vi "Get Value.vi"(8 "error in (no error)":errorcluster, 11 "Acquired Result in":refnum<class "Acquired Result.lvclass">) -> (0 "error out":errorcluster, 2 "Value":dynamicdata(graph) caption="Filtered Signal", 3 "Acquired Result out":refnum<class "Acquired Result.lvclass">)   [LabVIEW 2021, in "Acquired Result.lvclass"]
uses:
  Acquired Result.lvclass
  Acquired Result.lvclass/Acquired Result.ctl
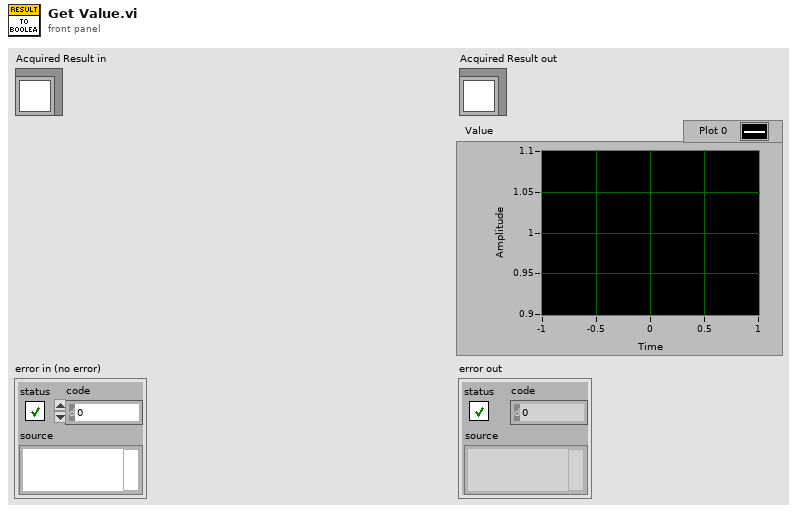
[diagram p1: front panel]
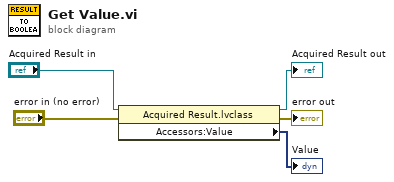
[diagram p0: block diagram]
diagram:
  n1 = property class="Acquired Result.lvclass"(reference="Acquired Result in", error in="error in (no error)") -> (reference out=→"Acquired Result out":refnum<class "Acquired Result.lvclass">, error out=→"error out":errorcluster, "Accessors:Value"=→"Value":dynamicdata)
